vi "TraverseControl.vi"(0 "Mode":T5=enum."Read traverse position", 1 "Work in Tunnel Coordinates?":T2, 2 "Probe Support":T1=[{"Max"=15001.0, "Min"=12000.0}, {"Max"=1000.0, "Min"=-1000.0}, {"Max"=700.0, "Min"=0.0}] {"Min" format="%#.1f"; "Max" format="%#.1f"}, 3 "Model       Roll      Pitch       Yaw (deg)":dbl[](array[numeric]) format="%#.2f", 4 "Probe Volume":T1=[{"Max"=15.0, "Min"=-15.0}, {"Max"=250.0, "Min"=0.0}, {"Max"=15.0, "Min"=-15.0}] {"Min" format="%#.1f"; "Max" format="%#.1f"}, 5 "Position input XYZ":dbl[](array[numeric])=[0.0, 0.0, 0.0] format="%.2f", 6 "Route Checking?":bool, 7 "Entire Space":T1=[{"Max"=15001.0, "Min"=12000.0}, {"Max"=1000.0, "Min"=-1000.0}, {"Max"=700.0, "Min"=0.0}] {"Min" format="%#.1f"; "Max" format="%#.1f"}, 10 "Exclude Array":T3[](array[typedef]) {"Sizes"."Min" format="%#.1f"; "Sizes"."Max" format="%#.1f"}, 11 "Speed Factor":dbl=1.0 min=0.1 max=5.0 format="%.2f", 12 "Traverse Name":string, 13 "Backlash Compensation?":bool=TRUE) -> (14 "Position Output XYZ":dbl[](array[numeric]) format="%.2f", 19 "Error String":string)   [LabVIEW 2013]
uses:
  Anemometry/Anemometry Sub Vis/Gen Trav/Trav_mode.ctl
  Anemometry/Anemometry Sub Vis/Gen Trav/Route mapping/Exclude_cluster.ctl
  Anemometry/Anemometry Sub Vis/Gen Trav/Route mapping/Box_size.ctl
  Anemometry/Anemometry Sub Vis/Gen Trav/Route mapping/Exclusion_type.ctl
  Anemometry/Anemometry Sub Vis/Controls/Tunnel_Coordinates.ctl
  ~subVIs/GenericDriveCommand.ctl
  ADAM Client/Sub VIs/ADAM Controls/Update_scan_value.ctl
  Anemometry/Anemometry Sub Vis/Globals/Trav_pos_global.vi
  Anemometry/Anemometry Sub Vis/Globals/Preference_global.vi
  ~subVIs/DriveConfigGlobal.vi
panel:
  out "Server copy Location":path
  out "Position Steps":dbl[][](array[numeric]) format="%.2f"
  out "Log File":path
  out "Achieved Pos In Eng units of all channels":dbl[](array[numeric]) format="%.2f"
  out "Pulses Positon all channels":dbl[](array[numeric])
  out "Counters Reset?":bool
  # "X                Y                   Z"
  # "X                           Y                          Z"
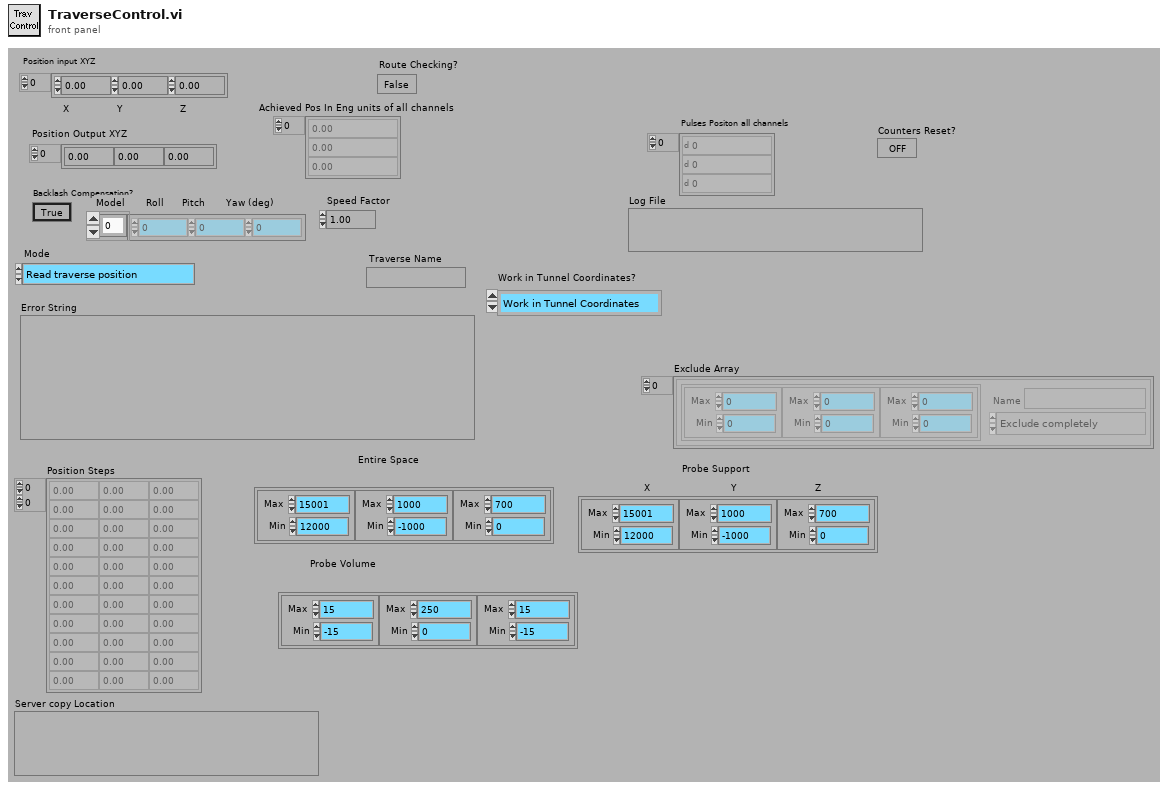
[diagram p1: front panel]
types:
  T1 = typedef "Box_size.ctl" = cluster{"Max":dbl, "Min":dbl}[]
  T2 = typedef "Tunnel_Coordinates.ctl" = enum16{"Work in Tunnel Coordinates", "Work in Model Coordinates"}
  T3 = typedef "Exclude_cluster.ctl" = cluster{"Sizes":T1, "Name":string, "Exclude Type":T4}
  T4 = typedef "Exclusion_type.ctl" = enum16{"Exclude completely", "Allow only vertical moves"}
  T5 = typedef "Trav_mode.ctl" = enum16{"Move traverse", "Read traverse position", "Teach Position"}
  T6 = typedef "GenericDriveCommand.ctl" = string
  T7 = enum16{"To Traverse Coordinates", "To User Coordinates"}
  T8 = typedef "Update_scan_value.ctl" = cluster{"Channel Name":string, "New Value":dbl}
  T9 = typedef "AxisConfigCluster.ctl" = cluster{"Channel Properties":T10, "Static Drive Configuration":T11}
  T10 = typedef "DriveProperties.ctl" = cluster{"Channel Name":string, "Vel. Default":dbl, "Acc. Default":dbl, "Vel. Max":dbl, "Vel. Min":dbl, "Acc. Max":dbl, "Acc. Min":dbl, "Pulses/unit":dbl, "Address":u8, "Pulse Offset":i32, "Pos Tolerance":dbl, "Pulses/rev":dbl, "Backlash/Eng units":dbl, "Current Pos":dbl, "Ch Status":enum16{"Active", "Offline", "Simulate"}, "Port Name":string, "Axis Transform mode":string, "Metadata Ch Name":string, "Type":string}
  T11 = typedef "DriveStaticConfig.ctl" = cluster{"Correction Gain % (CG)":u16, "Dead Band (DB)":i32, "Dead Band Window (DW)":i32, "Encoder Resolution (ER)":i32, "Step Mode  (FSB)":u16, "Position Maintenance (FSC)":u16, "Stop on Stall (FSD)":u16, "Activate OP1 on stall (FSE)":u16, "Stop on Trigger 3 (FSF)":u16, "OP2 in Deadband (FSG)":u16, "Stall Detect (FSH)":u16, "Limit Disable (LD)":u16, "Motor Resolution (MR)":enum16{"200", "400", "1000", "2000", "4000", "5000", "10000", "12800", "18000", "20000", "21600", "25000", "25400", "25600", "36000", "50000", "278528", "425984", "507904", "614400", "655360", "819200", "1024000"}, "Limit Switch Sense (OSA)":u16, "Home Position (OSB)":u16, "Home Switch Sense (OSC)":u16, "Encoder Z for Home (OSD)":u16, "Reference edge of Home (OSH)":u16, "RS232 Echo Control (SSA)":u16, "Buffer at Limit (SSG)":u16, "Buffer at Stop (SSH)":u16, "Indexer Mode  (FSA)":u16, "Type":string, "ConfigString":string, "De Power Motor":enum16{"TRUE", "FALSE"}}
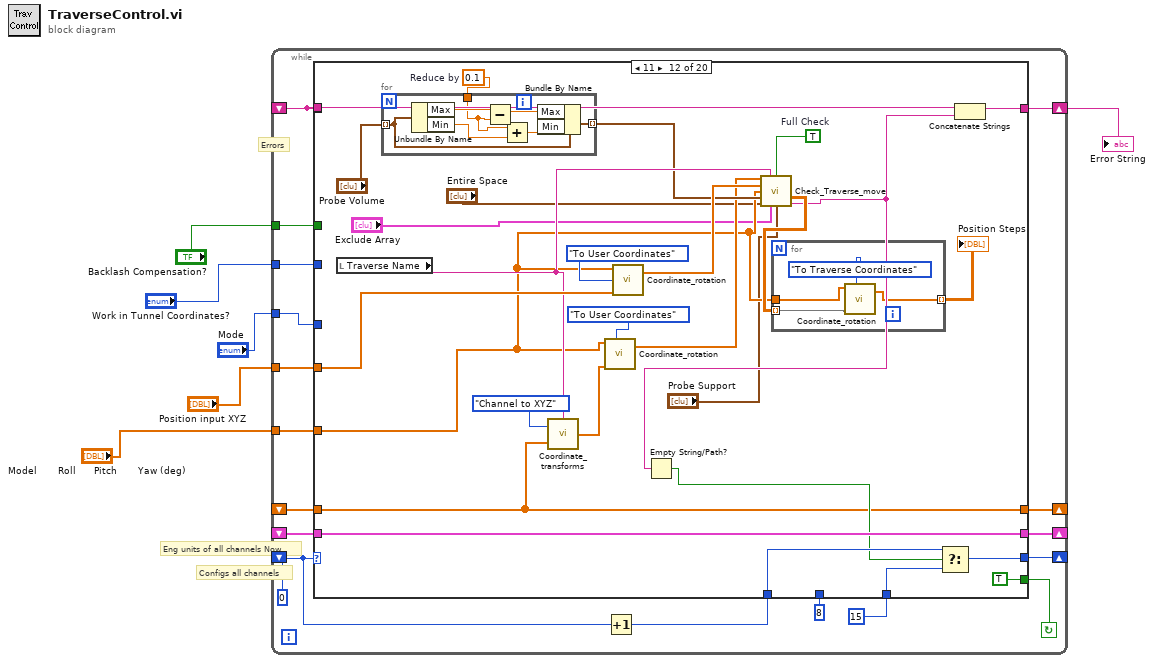
[diagram p0: block diagram]
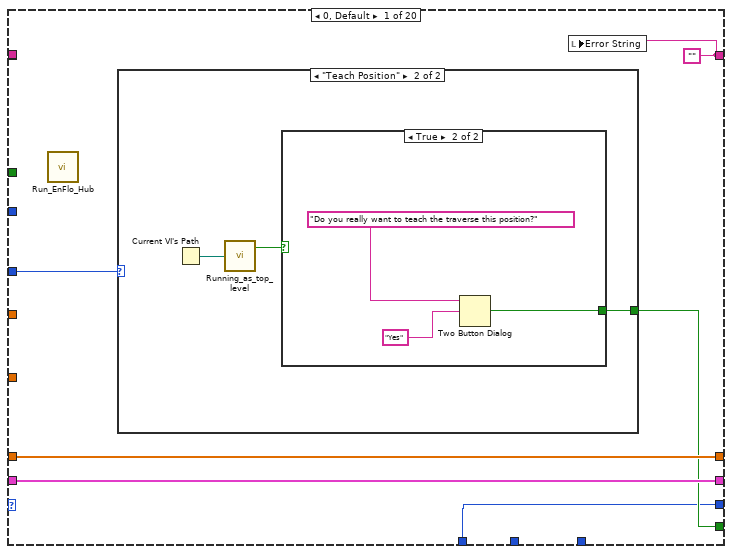
[diagram p2: hidden frame]
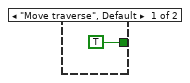
[diagram p3: hidden frame]
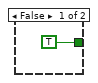
[diagram p4: hidden frame]
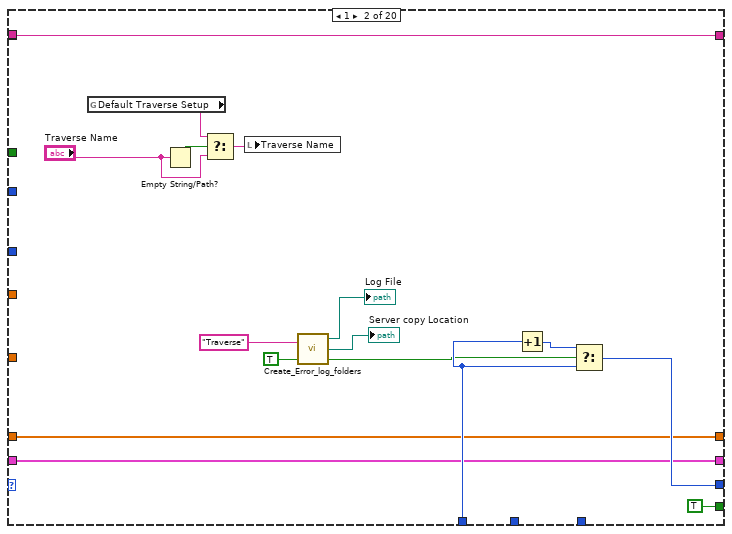
[diagram p5: hidden frame]
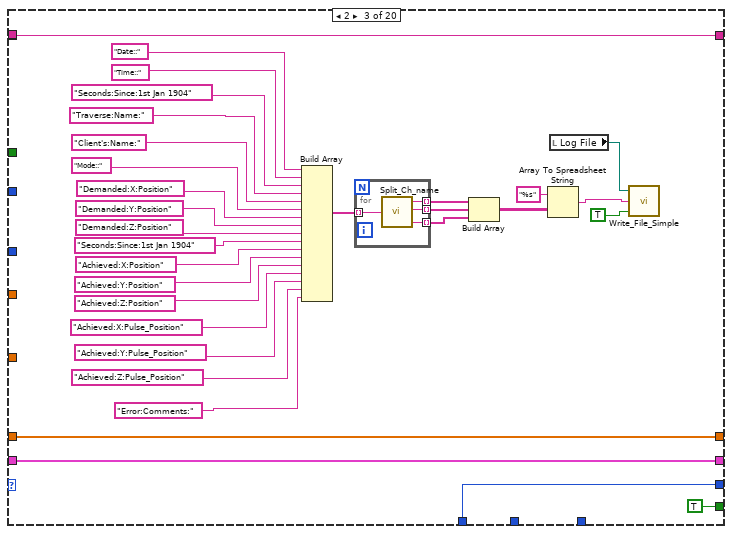
[diagram p6: hidden frame]
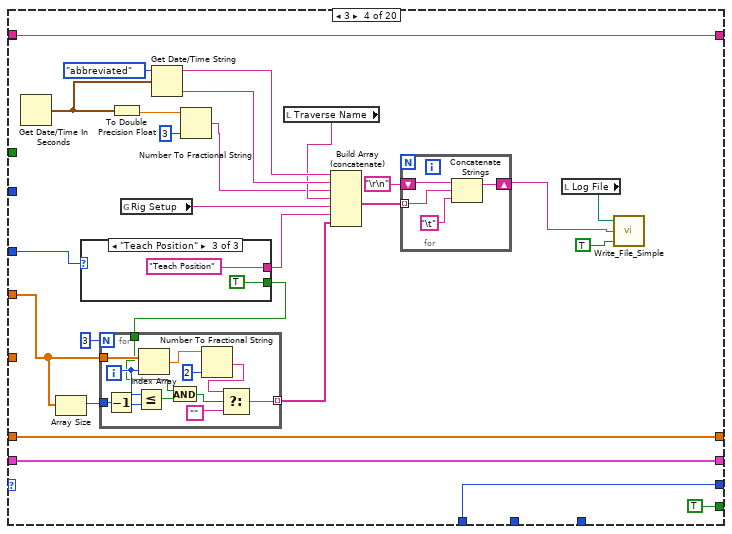
[diagram p7: hidden frame]
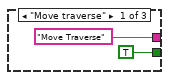
[diagram p8: hidden frame]
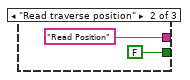
[diagram p9: hidden frame]
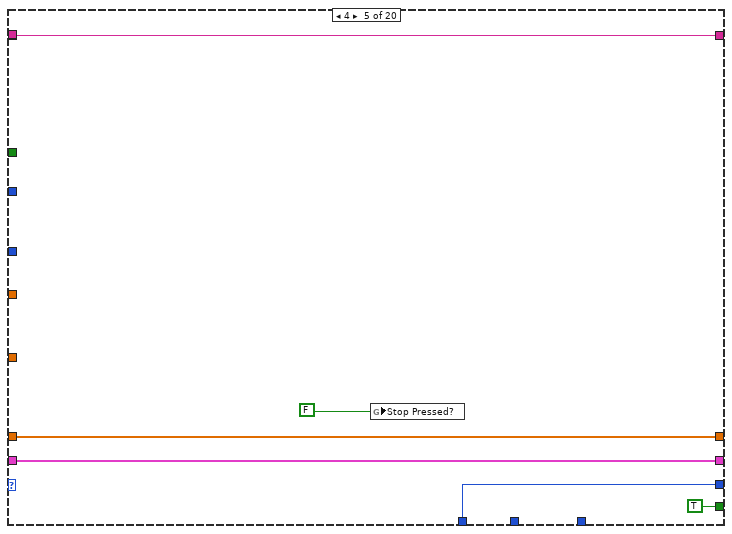
[diagram p10: hidden frame]
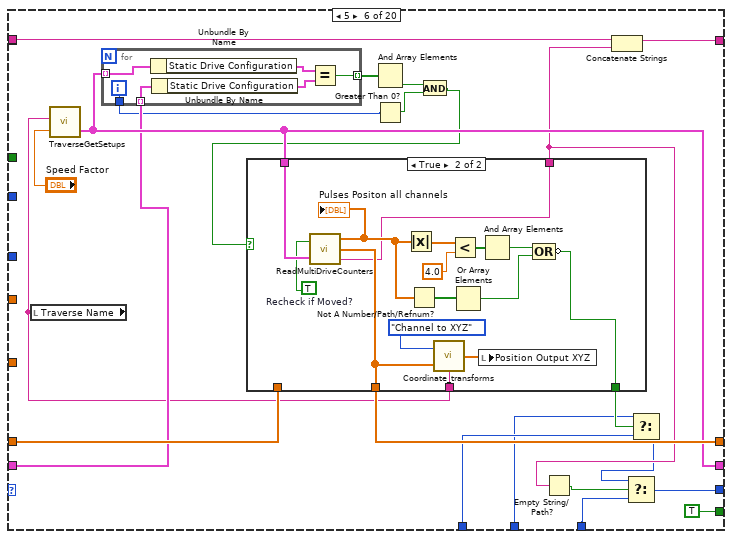
[diagram p11: hidden frame]
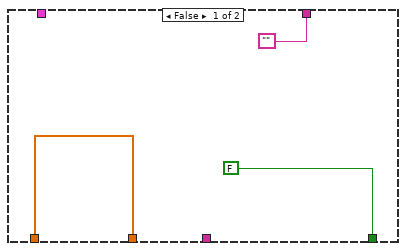
[diagram p12: hidden frame]
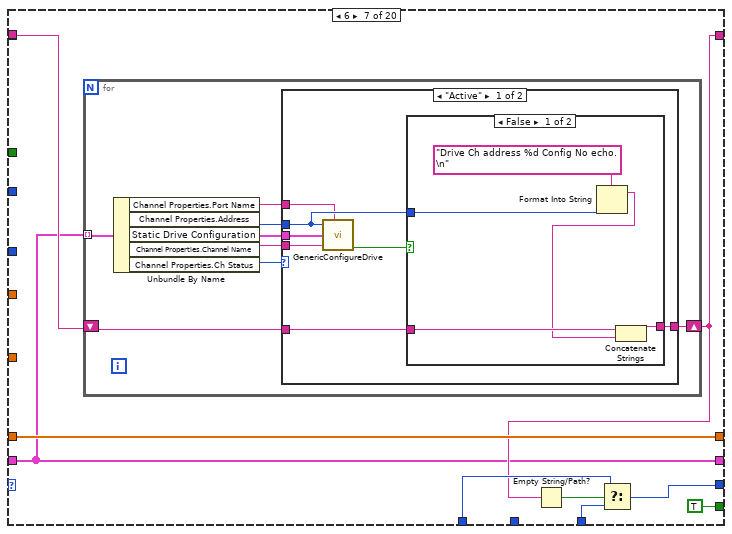
[diagram p13: hidden frame]
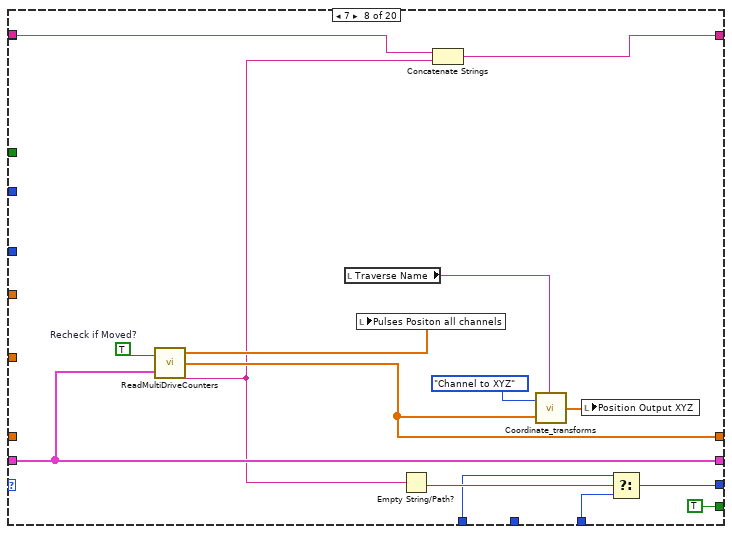
[diagram p16: hidden frame]
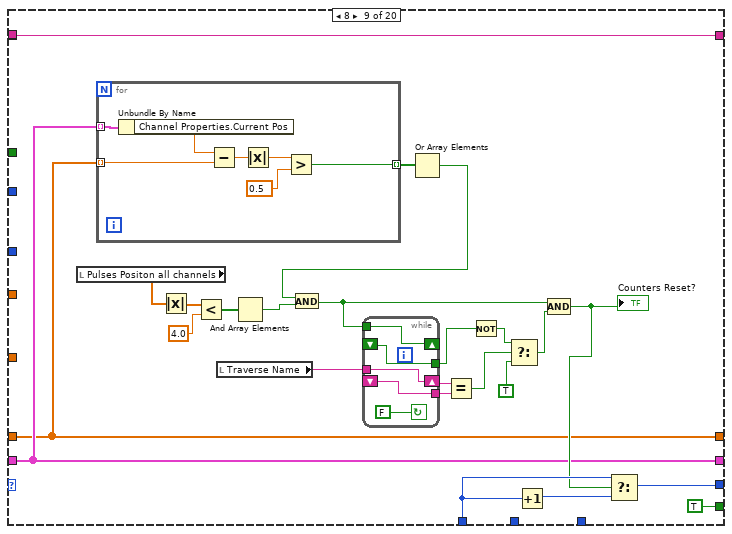
[diagram p17: hidden frame]
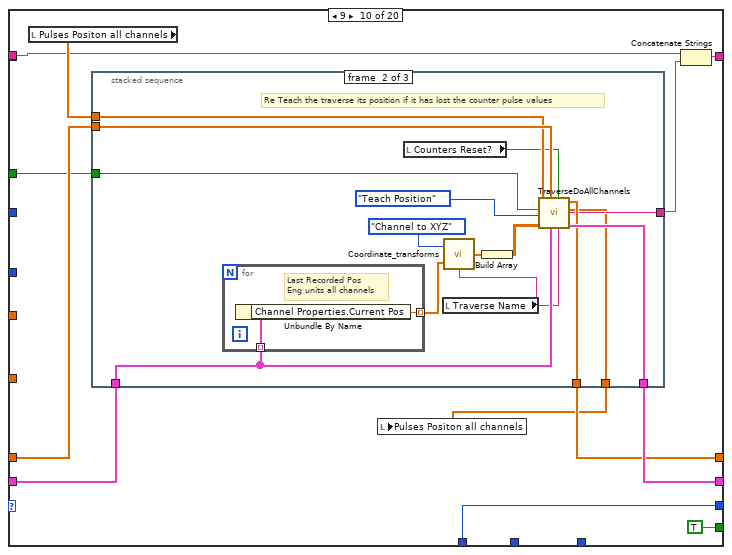
[diagram p18: hidden frame]
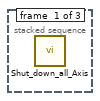
[diagram p19: hidden frame]
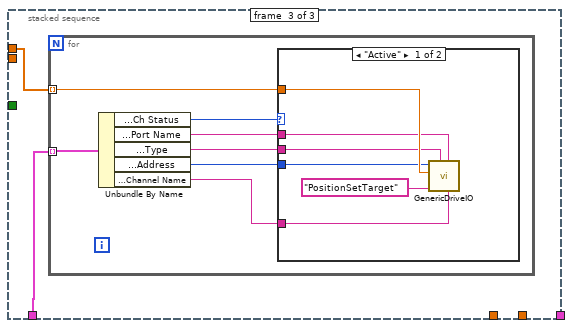
[diagram p20: hidden frame]
diagram:
  # "Errors"
  # "Eng units of all channels Now"
  # "Configs all channels"
  n1 = while {
    tunnel: "Backlash Compensation?" -> [w10]
    tunnel: "Position input XYZ" -> [w14]
    shift-left: _ -> [w11]
    shift-right: [w15] -> w5
    shift-left: _ -> [w16]
    shift-right: [w17] -> _
    shift-left: _ -> [w18]
    shift-right: [w19] -> _
    shift-left: 0 -> [w22]
    shift-right: [w20] -> _
    tunnel: "Mode" -> [w24]
    tunnel: "Model       Roll      Pitch       Yaw (deg)" -> [w9]
    tunnel: "Work in Tunnel Coordinates?" -> [w8]
    stop <- w23 continue-if-true
    n2 = Increment(x=w22) -> (x+1=w21:i32)
    n3 = case shown="11" w22 {
      tunnel: w24 -> [w30 _ _ w108 _ _ _ _ _ _ w323 _ w389 w396 _ _ _ w471 _ w527]
      tunnel: [w27 TRUE ("T button?") TRUE ("T button?") TRUE ("T button?") TRUE TRUE ("T button?") TRUE ("T button?") TRUE ("T button?") TRUE TRUE TRUE ("T button?") TRUE ("T button?") TRUE TRUE TRUE ("T button?") TRUE ("T button?") TRUE ("T button?") w473 TRUE FALSE] -> w23
      tunnel: w21 -> [w26 w53 w65 w113 w138 w162 w195 w223 w255 w274 w322 w357 w380 w398 w421 w438 w466 w470 w505 w534]
      tunnel: [w26 w51 w65 w113 w138 w145 w194 w221 w253 w274 w321 w358 w380 w397 w421 w436 w466 w469 w505 w534] -> w20
      tunnel: [w28 w48 w67 w115 w140 w160 w190 w235 w250 w283 w319 w360 w373 w395 w423 w449 w468 w476 w503 w532] -> w19
      tunnel: w18 -> [w28 w48 w67 w115 w140 w159 w190 w235 w250 w282 w319 w360 w387 w395 w423 w449 w468 w476 w503 w532]
      tunnel: [w29 w49 w66 w114 w141 w165 w198 w230 w249 w279 w318 w347 w381 w401 w422 w448 w467 w477 w506 w535] -> w17
      tunnel: w16 -> [w29 w49 w66 w114 w141 w164 w198 _ w249 w280 w318 w347 w376 w401 w422 w448 w467 w477 w506 w535]
      tunnel: [w25 w47 w63 w105 w142 w150 w191 w226 w252 w276 w324 w351 w383 w399 w419 w440 w464 w472 w499 w528] -> w15
      tunnel: w11 -> [_ w47 w63 w105 w142 w151 w192 w227 w252 w278 w324 _ w384 w399 w419 w440 w464 w475 w501 w530]
      tunnel: w14 -> [_ _ _ w102 _ _ _ _ _ _ w317 w349 _ _ _ _ _ _ w497 _]
      tunnel: 15 ("f") -> [_ _ _ _ _ w146 w193 w222 _ _ _ w353 _ _ _ _ _ _ _ _]
      tunnel: 8 ("t") -> [_ _ _ _ _ w161 _ _ _ _ _ _ _ _ _ _ _ _ _ _]
      tunnel: w11 -> [_ _ _ _ _ _ _ _ _ _ _ w354 _ _ _ _ _ _ _ _]
      tunnel: w10 -> [_ _ _ _ _ _ _ _ _ w273 _ _ w375 _ _ _ _ _ _ _]
      tunnel: w9 -> [_ _ _ _ _ _ _ _ _ _ _ w337 _ _ _ _ _ _ w498 w525]
      tunnel: w8 -> [_ _ _ _ _ _ _ _ _ _ _ _ _ _ _ _ _ _ w495 w523]
      frame 0, Default {
        w25 = ""
        n4 = call "Run_EnFlo_Hub.vi"() -> ()  [unwired: 8 out]
        n5 = case shown="\"Teach Position\"" w30 {
          tunnel: [TRUE ("T button?") w32] -> w27
          frame "Move traverse", Default {
          }
          frame "Teach Position" {
            n6 = Current VI's Path() -> (path=w34:path)
            n7 = call "Running_as_top_level.vi"("Vi path name"=w34) -> ("Top Level"=w33:bool)  [unwired: 1 out]
            n8 = case shown="True" w33 {
              tunnel: [TRUE ("T button?") w36] -> w32
              frame False {
              }
              frame True {
                n9 = Two Button Dialog(message="Do you really want to teach the traverse this position?", 2:"Yes" ("T button name (\"OK\")")) -> (T button?=w36:bool)  [unwired: 1 out]
              }
            }
          }
        }
        n10 = local write "Error String"(w25) -> ()
      }
      frame 1 {
        n11 = global read "Trav_pos_global.vi" "Default Traverse Setup"() -> (w44:string)
        n12 = Empty String/Path?(string/path="Traverse Name") -> (empty?=w42:bool)
        n13 = Select(t=w44, s=w42, f="Traverse Name") -> (s? t:f=w41:string)
        n14 = local write "Traverse Name"(w41) -> ()
        n15 = call "Create_Error_log_folders.vi"("Per Day Log File?"=TRUE, "Log Filename"="Traverse" ("Input Element")) -> ("exists?"=w45:bool, "Server copy Location"=→"Server copy Location":path, "Local Log File"=→"Log File":path)  [unwired: 1 in]
        n16 = Increment(x=w53) -> (x+1=w52:i32)
        n17 = Select(t=w52, s=w45, f=w53) -> (s? t:f=w51:i32)
      }
      frame 2 {
        n18 = Build Array("Date::", "Time::", "Seconds:Since:1st Jan 1904", "Traverse:Name:", "Client's:Name:", "Mode::", "Demanded:X:Position", "Demanded:Y:Position", "Demanded:Z:Position", "Seconds:Since:1st Jan 1904", "Achieved:X:Position", "Achieved:Y:Position", "Achieved:Z:Position", "Achieved:X:Pulse_Position", "Achieved:Y:Pulse_Position", "Achieved:Z:Pulse_Position", "Error:Comments:") -> (w70:string[])
        n19 = for {
          tunnel: w70 -> [w89] mode=indexing
          tunnel: [w88] -> w71 mode=indexing
          tunnel: [w87] -> w72 mode=indexing
          tunnel: [w86] -> w73 mode=indexing
          n20 = call "Split_Ch_name.vi"("Ch name"=w89) -> ("Top level"=w88:string, "Middle"=w87:string, "Low level"=w86:string)
        }
        n21 = Build Array(w71, w72, w73) -> (w68:string[][])
        n22 = Array To Spreadsheet String(array=w68, 3:"%s" ("format string")) -> (spreadsheet string=w61:string)  [unwired: 1 out]
        n23 = local read "Log File"() -> (w60:path)
        n24 = call "Write_File_Simple.vi"("append to file? (new file:F)"=TRUE, "character string"=w61, "file path"=w60) -> ()  [unwired: 2 out]
      }
      frame 3 {
        n25 = Get Date/Time In Seconds() -> (seconds since 1Jan1904=w94:timestamp)
        n26 = Array Size(array=w102) -> (size(s)=w103:i32)
        n27 = case shown="\"Teach Position\"" w108 {
          tunnel: ["Move Traverse" "Read Position" "Teach Position"] -> w109
          tunnel: [TRUE FALSE TRUE] -> w99
          frame "Move traverse" {
          }
          frame "Read traverse position" {
          }
          frame "Teach Position" {
          }
        }
        n28 = for {
          N: 3 -> [_]
          tunnel: w102 -> [w127]
          tunnel: w103 -> [w124]
          tunnel: [w120] -> w100 mode=indexing
          tunnel: w99 -> [w116]
          i -> [w122]
          n29 = Decrement(x=w124) -> (x-1=w123:i32)
          n30 = Less Or Equal?(x=w122, y=w123) -> (x <= y?=w118:bool)
          n31 = Index Array(array=w127, index=w122) -> (element=w126:dbl)
          n32 = And(x=w116, y=w118) -> (x .and. y?=w117:bool)
          n33 = Number To Fractional String(number=w126, precision (6)=i16 2) -> (F-format string=w121:string)  [unwired: 2 out]
          n34 = Select(t=w121, s=w117, f="") -> (s? t:f=w120:string)
        }
        n35 = To Double Precision Float(number=w94) -> (double precision float=w93:dbl)
        n36 = global read "Preference_global.vi" "Rig Setup"() -> (w90:string)
        n37 = Get Date/Time String(date format (0)=enum16{"short", "long", "abbreviated"}."abbreviated", seconds (now)=w94) -> (date string=w111:string, time string=w110:string)  [unwired: 1 out]
        n38 = Number To Fractional String(number=w93, precision (6)=i16 3) -> (F-format string=w91:string)  [unwired: 2 out]
        n39 = local read "Traverse Name"() -> (w95:string)
        n40 = Build Array (concatenate)(w111, w110, w91, w95, w90, w109, w100) -> (w106:string[])
        n41 = for {
          shift-right: [w130] -> w96
          shift-left: "\r\n" -> [w131]
          tunnel: w106 -> [w129] mode=indexing
          n42 = Concatenate Strings(w131, w129, "\t") -> (w130:string)
        }
        n43 = local read "Log File"() -> (w97:path)
        n44 = call "Write_File_Simple.vi"("append to file? (new file:F)"=TRUE, "character string"=w96, "file path"=w97) -> ()  [unwired: 2 out]
      }
      frame 4 {
        n45 = global write "DriveConfigGlobal.vi" "Stop Pressed?"(FALSE) -> ()
      }
      frame 5 {
        n46 = local read "Traverse Name"() -> (w153:string)
        n47 = call "TraverseGetSetups.vi"("Speed Factor"="Speed Factor", "Traverse Name"=w153) -> ("Matched Configurations"=w160:T9[])  [unwired: 1 out]
        n48 = for {
          tunnel: w160 -> [w171] mode=indexing
          tunnel: w159 -> [w170] mode=indexing
          tunnel: [w167] -> w158 mode=indexing
          tunnel: [w166] -> w157
          i -> [w166]
          n49 = Unbundle By Name(w171) -> ("Static Drive Configuration"=w169:T11)
          n50 = Unbundle By Name(w170) -> ("Static Drive Configuration"=w168:T11)
          n51 = Equal?(x=w169, y=w168) -> (x = y?=w167:bool)
        }
        n52 = And Array Elements(Boolean array=w158) -> (logical AND=w155:bool)
        n53 = Greater Than 0?(x=w157) -> (x > 0?=w156:bool)
        n54 = And(x=w155, y=w156) -> (x .and. y?=w154:bool)
        n55 = case shown="True" w154 {
          tunnel: w160 -> [_ w189]
          tunnel: [w174 w179] -> w165
          tunnel: w164 -> [w174 _]
          tunnel: [FALSE w181] -> w163
          tunnel: w153 -> [_ w177]
          tunnel: ["" w175] -> w149
          frame False {
          }
          frame True {
            w176 = TRUE  # Recheck if Moved?
            n56 = call "ReadMultiDriveCounters.vi"("Recheck if Moved?"=w176, "Matched Configurations"=w189) -> ("Pulses"=w184:dbl[], "Eng units"=w179:dbl[], "Error String"=w175:string)
            "Pulses Positon all channels" <- w184
            n57 = Absolute Value(x=w184) -> (abs(x)=w188:dbl[])
            n58 = Not A Number/Path/Refnum?(number/path/refnum=w184) -> (NaN/Path/Refnum?=w183:bool[])
            n59 = call "Coordinate_transforms.vi"("Traverse Name"=w177, "Input"=w179, "Mode"=enum16{"XYZ to Channel", "Channel to XYZ"}."Channel to XYZ") -> ("Output"=w178:dbl[])
            n60 = Less?(x=w188, y=4.0 ("Achieved Position")) -> (x < y?=w186:bool[])
            n61 = Or Array Elements(Boolean array=w183) -> (logical OR=w182:bool)
            n62 = local write "Position Output XYZ"(w178) -> ()
            n63 = And Array Elements(Boolean array=w186) -> (logical AND=w185:bool)
            n64 = Compound Arithmetic op=OR(w185, w182) -> (invert w181:bool)
          }
        }
        n65 = Empty String/Path?(string/path=w149) -> (empty?=w148:bool)
        n66 = Concatenate Strings(w151, w149) -> (w150:string)
        n67 = Select(t=w161, s=w163, f=w162) -> (s? t:f=w147:i32)
        n68 = Select(t=w147, s=w148, f=w146) -> (s? t:f=w145:i32)
      }
      frame 6 {
        n69 = for {
          tunnel: w190 -> [w206] mode=indexing
          shift-right: [w199] -> w191
          shift-left: w192 -> [w200]
          n70 = Unbundle By Name(w206) -> ("Channel Properties.Port Name"=w201:string, "Channel Properties.Address"=w205:u8, "Static Drive Configuration"=w204:T11, "Channel Properties.Channel Name"=w203:string, "Channel Properties.Ch Status"=w202:enum16{"Active", "Offline", "Simulate"})
          n71 = case shown="\"Active\"" w202 {
            tunnel: w205 -> [w211 _]
            tunnel: w204 -> [w213 _]
            tunnel: w203 -> [w212 _]
            tunnel: w201 -> [w210 _]
            tunnel: w200 -> [w208 w220]
            tunnel: [w207 w220] -> w199
            frame "Active" {
              n72 = call "GenericConfigureDrive.vi"("Address"=w211, "Port Name"=w210, "Static Drive Configuration"=w213, "Channel Name"=w212) -> ("Good Echo"=w209:bool)  [unwired: 4 out]
              n73 = case shown="False" w209 {
                tunnel: w211 -> [w218 _]
                tunnel: w208 -> [w216 w219]
                tunnel: [w215 w219] -> w207
                frame False {
                  n74 = Format Into String(format string="Drive Ch address %d Config No echo.\n" ("Format String"), w218) -> (resulting string=w214:string)  [unwired: 2 in, 1 out]
                  n75 = Concatenate Strings(w216, w214) -> (w215:string)
                }
                frame True {
                }
              }
            }
            frame "Offline", Default {
            }
          }
        }
        n76 = Empty String/Path?(string/path=w191) -> (empty?=w196:bool)
        n77 = Select(t=w195, s=w196, f=w193) -> (s? t:f=w194:i32)
      }
      frame 7 {
        w228 = TRUE  # Recheck if Moved?
        n78 = call "ReadMultiDriveCounters.vi"("Recheck if Moved?"=w228, "Matched Configurations"=w235) -> ("Pulses"=w233:dbl[], "Eng units"=w230:dbl[], "Error String"=w224:string)
        n79 = local read "Traverse Name"() -> (w229:string)
        n80 = local write "Pulses Positon all channels"(w233) -> ()
        n81 = Empty String/Path?(string/path=w224) -> (empty?=w225:bool)
        n82 = Concatenate Strings(w227, w224) -> (w226:string)
        n83 = call "Coordinate_transforms.vi"("Traverse Name"=w229, "Input"=w230, "Mode"=enum16{"XYZ to Channel", "Channel to XYZ"}."Channel to XYZ") -> ("Output"=w231:dbl[])
        n84 = local write "Position Output XYZ"(w231) -> ()
        n85 = Select(t=w223, s=w225, f=w222) -> (s? t:f=w221:i32)
      }
      frame 8 {
        n86 = local read "Pulses Positon all channels"() -> (w244:dbl[])
        n87 = for {
          tunnel: w250 -> [w271] mode=indexing
          tunnel: w249 -> [w269] mode=indexing
          tunnel: [w265] -> w247 mode=indexing
          n88 = Unbundle By Name(w271) -> ("Channel Properties.Current Pos"=w270:dbl)
          n89 = Subtract(x=w270, y=w269) -> (x-y=w268:dbl)
          n90 = Absolute Value(x=w268) -> (abs(x)=w267:dbl)
          n91 = Greater?(x=w267, y=0.5) -> (0:w265:bool)
        }
        n92 = Absolute Value(x=w244) -> (abs(x)=w259:dbl[])
        n93 = Less?(x=w259, y=4.0 ("Achieved Position")) -> (x < y?=w257:bool[])
        n94 = local read "Traverse Name"() -> (w243:string)
        n95 = And Array Elements(Boolean array=w257) -> (logical AND=w248:bool)
        n96 = Or Array Elements(Boolean array=w247) -> (logical OR=w246:bool)
        n97 = And(x=w246, y=w248) -> (x .and. y?=w245:bool)
        n98 = while {
          tunnel: [w263] -> w237
          tunnel: w245 -> [w264]
          shift-left: _ -> [w263]
          shift-right: [w264] -> _
          shift-right: [w261] -> w242
          shift-left: _ -> [w260]
          tunnel: w243 -> [w261]
          tunnel: [w260] -> w241
          stop <- FALSE continue-if-true
        }
        n99 = Equal?(x=w242, y=w241) -> (x = y?=w240:bool)
        n100 = Not(x=w237) -> (.not. x?=w236:bool)
        n101 = Select(t=w236, s=w240, f=TRUE) -> (s? t:f=w239:bool)
        n102 = Increment(x=w255) -> (x+1=w254:i32)
        n103 = Compound Arithmetic op=AND(w245, w239) -> (w251:bool)
        "Counters Reset?" <- w251
        n104 = Select(t=w255, s=w251, f=w254) -> (s? t:f=w253:i32)
      }
      frame 9 {
        n105 = local read "Pulses Positon all channels"() -> (w281:dbl[])
        n106 = stacked-sequence {
          tunnel: w281 -> [_ w290 w301]
          tunnel: [_ w298 _] -> w283
          tunnel: w280 -> [_ w297 _]
          tunnel: [_ w296 _] -> w279
          tunnel: w282 -> [_ w292 w302]
          tunnel: [_ w295 _] -> w277
          tunnel: w273 -> [_ w286 _]
          tunnel: [_ w284 _] -> w272
          frame #0 {
            n107 = call "Shut_down_all_Axis.vi"() -> ()  [unwired: 1 out]
          }
          frame #1 {
            # "Re Teach the traverse its position if it has lost the counter pulse values"
            n108 = for {
              tunnel: [w300] -> w291 mode=indexing
              tunnel: w292 -> [w299] mode=indexing
              # "Last Recorded Pos\nEng units all channels"
              n109 = Unbundle By Name(w299) -> ("Channel Properties.Current Pos"=w300:dbl)
            }
            n110 = local read "Counters Reset?"() -> (w288:bool)
            n111 = local read "Traverse Name"() -> (w287:string)
            n112 = call "Coordinate_transforms.vi"("Traverse Name"=w287, "Input"=w291, "Mode"=enum16{"XYZ to Channel", "Channel to XYZ"}."Channel to XYZ") -> ("Output"=w293:dbl[])
            n113 = Build Array(w293) -> (w285:dbl[][])
            n114 = call "TraverseDoAllChannels.vi"("Traverse Name"=w287, "Counters Reset?"=w288, "Matched Configurations all Channels In"=w292, "Current Pos In Eng units of all channels"=w297, "Position Steps"=w285, "Mode"=Trav_mode."Teach Position", "Backlash Compensation?"=w286, "Current Pulses positions for all channels"=w290) -> ("Matched Configurations Out"=w298:T9[], "Error String"=w295:string, "Current Pulses positions for all channels Out"=w284:dbl[], "Achieved Pos In Eng units of all channels"=w296:dbl[])
          }
          frame #2 {
            n115 = for {
              tunnel: w302 -> [w309] mode=indexing
              tunnel: w301 -> [w308] mode=indexing
              n116 = Unbundle By Name(w309) -> ("Channel Properties.Ch Status"=w307:enum16{"Active", "Offline", "Simulate"}, "Channel Properties.Port Name"=w306:string, "Channel Properties.Type"=w305:string, "Channel Properties.Address"=w304:u8, "Channel Properties.Channel Name"=w303:string)
              n117 = case shown="\"Active\"" w307 {
                tunnel: w308 -> [w315 _]
                tunnel: w306 -> [w314 _]
                tunnel: w305 -> [w313 _]
                tunnel: w304 -> [w312 _]
                tunnel: w303 -> [w311 _]
                frame "Active" {
                  n118 = call "GenericDriveIO.vi"("GenericDriveCommand"=T6 "PositionSetTarget", "Channel Name"=w311, "Numeric Value"=w315, "Address"=w312, "Type"=w313, "Port Name"=w314) -> ()  [unwired: 1 in, 5 out]
                }
                frame "Offline", Default {
                }
              }
            }
          }
        }
        n119 = local write "Pulses Positon all channels"(w272) -> ()
        n120 = Concatenate Strings(w278, w277) -> (w276:string)
      }
      frame 10 {
        n121 = Build Array(w317) -> (w316:dbl[][])
        n122 = local write "Position Steps"(w316) -> ()
        n123 = case shown="\"Read traverse position\", Default" w323 {
          tunnel: w322 -> [w325 w332]
          tunnel: [w327 w331] -> w321
          frame "Move traverse" {
            n124 = Increment(x=w325) -> (x+1=w326:i32)
            n125 = case shown="True" "Route Checking?" {
              tunnel: [w329 w330] -> w327
              tunnel: w326 -> [w329 _]
              tunnel: w325 -> [_ w330]
              frame False {
              }
              frame True {
              }
            }
          }
          frame "Read traverse position", Default {
            n126 = Increment(x=w332) -> (x+1=w331:i32)
          }
        }
      }
      frame 11 {
        w342 = 0.1  # Reduce by
        w346 = TRUE  # Full Check
        n127 = local read "Traverse Name"() -> (w348:string)
        n128 = for {
          tunnel: "Probe Volume" -> [w367] mode=indexing
          tunnel: [w366] -> w341 mode=indexing
          tunnel: w342 -> [w361]
          n129 = Unbundle By Name(w367) -> ("Max"=w365:dbl, "Min"=w363:dbl)
          n130 = Subtract(x=w365, y=w361) -> (x-y=w364:dbl)
          n131 = Add(x=w361, y=w363) -> (x+y=w362:dbl)
          n132 = Bundle By Name(cluster=w367, "Max"=w364, "Min"=w362) -> (w366:cluster{"Max":dbl, "Min":dbl})
        }
        n133 = call "Coordinate_transforms.vi"("Traverse Name"=w348, "Input"=w347, "Mode"=enum16{"XYZ to Channel", "Channel to XYZ"}."Channel to XYZ") -> ("Output"=w339:dbl[])
        n134 = call "Coordinate_rotation.vi"("Model       Roll      Pitch       Yaw (deg)"=w337, "Input Position"=w339, "Mode"=T7."To User Coordinates") -> ("Output Position"=w338:dbl[])  [unwired: 2 in, 1 out]
        n135 = call "Coordinate_rotation.vi"("Model       Roll      Pitch       Yaw (deg)"=w337, "Input Position"=w349, "Mode"=T7."To User Coordinates") -> ("Output Position"=w355:dbl[])  [unwired: 2 in, 1 out]
        n136 = call "Check_Traverse_move.vi"("Current position"=w338, "Traverse Name"=w348, "Full Check"=w346, "New Position"=w355, "Model       Roll      Pitch       Yaw (deg)"=w337, "Probe Volume"=w341, "Entire Space"="Entire Space", "Exclude Array"="Exclude Array", "Probe Support"="Probe Support") -> ("Steps"=w345:dbl[][], "Error Comments"=w343:string)  [unwired: 5 out]
        n137 = Empty String/Path?(string/path=w343) -> (empty?=w352:bool)
        n138 = for {
          tunnel: w345 -> [w370] mode=indexing
          tunnel: [w369] -> w344 mode=indexing
          tunnel: w337 -> [w368]
          n139 = call "Coordinate_rotation.vi"("Model       Roll      Pitch       Yaw (deg)"=w368, "Input Position"=w370, "Mode"=T7."To Traverse Coordinates") -> ("Output Position"=w369:dbl[])  [unwired: 2 in, 1 out]
        }
        "Position Steps" <- w344
        n140 = Select(t=w357, s=w352, f=w353) -> (s? t:f=w358:i32)
        n141 = Concatenate Strings(w354, w343) -> (w351:string)
      }
      frame 12 {
        w378 = FALSE  # Counters Reset?
        n142 = local read "Pulses Positon all channels"() -> (w388:dbl[])
        n143 = local read "Traverse Name"() -> (w377:string)
        n144 = local read "Position Steps"() -> (w374:dbl[][])
        n145 = call "TraverseDoAllChannels.vi"("Traverse Name"=w377, "Counters Reset?"=w378, "Matched Configurations all Channels In"=w387, "Current Pos In Eng units of all channels"=w376, "Position Steps"=w374, "Mode"=w389, "Backlash Compensation?"=w375, "Current Pulses positions for all channels"=w388) -> ("Matched Configurations Out"=w373:T9[], "Error String"=w382:string, "Current Pulses positions for all channels Out"=w372:dbl[], "Achieved Pos In Eng units of all channels"=w381:dbl[])
        "Achieved Pos In Eng units of all channels" <- w381
        n146 = call "Coordinate_transforms.vi"("Traverse Name"=w377, "Input"=w381, "Mode"=enum16{"XYZ to Channel", "Channel to XYZ"}."Channel to XYZ") -> ("Output"=→"Position Output XYZ":dbl[])
        n147 = local write "Pulses Positon all channels"(w372) -> ()
        n148 = Concatenate Strings(w384, w382) -> (w383:string)
      }
      frame 13 {
        n149 = local read "Position Output XYZ"() -> (w393:dbl[])
        n150 = case shown="\"Teach Position\"" w396 {
          tunnel: w393 -> [_ w417 _]
          frame "Move traverse" {
          }
          frame "Read traverse position" {
            n151 = local write "Position input XYZ"(w417) -> ()
          }
          frame "Teach Position" {
            n152 = local write "Mode"(Trav_mode."Teach Position" ("Mode")) -> ()
          }
        }
        n153 = for {
          tunnel: w395 -> [w409] mode=indexing
          tunnel: T8 {"Channel Name"="", "New Value"=0.0} ("Update Scan Value Cluster") -> [w408]
          tunnel: w393 -> [w406] mode=indexing
          shift-right: [w404] -> w391
          shift-left: T8[] [] -> [w405]
          n154 = Unbundle By Name(w409) -> ("Channel Properties.Metadata Ch Name"=w407:string)
          n155 = Empty String/Path?(string/path=w407) -> (empty?=w403:bool)
          n156 = case shown="False" w403 {
            tunnel: w408 -> [w415 _]
            tunnel: w407 -> [w414 _]
            tunnel: w406 -> [w413 _]
            tunnel: w405 -> [w411 w416]
            tunnel: [w410 w416] -> w404
            frame False {
              n157 = Bundle By Name(cluster=w415, "Channel Name"=w414, "New Value"=w413) -> (w412:T8)
              n158 = Build Array (concatenate)(w411, w412) -> (w410:T8[])
            }
            frame True {
            }
          }
        }
        n159 = global write "DriveConfigGlobal.vi" "Run Emergency stop loop"(FALSE ("Run Emergency stop loop")) -> ()
        n160 = Increment(x=w398) -> (x+1=w397:i32)
        n161 = call "Update_Current_Value_client.vi"("Don't Bother with check?"=FALSE, "Update array in"=w391) -> ()
      }
      frame 14 {
      }
      frame 15 {
        n162 = local read "Pulses Positon all channels"() -> (w426:dbl[])
        n163 = local read "Position Output XYZ"() -> (w425:dbl[])
        n164 = Get Date/Time In Seconds() -> (seconds since 1Jan1904=w435:timestamp)
        n165 = To Double Precision Float(number=w435) -> (double precision float=w428:dbl)
        n166 = Number To Fractional String(number=w428, precision (6)=i16 3) -> (F-format string=w427:string)  [unwired: 2 out]
        n167 = call "Remove_unprintable_Char.vi"("Input String"=w440) -> ("Output String"=w441:string)
        n168 = Build Array (concatenate)(w425, w426) -> (w424:dbl[])
        n169 = Array Size(array=w424) -> (size(s)=w443:i32)
        n170 = for {
          N: 6 -> [_]
          tunnel: w424 -> [w463]
          tunnel: w443 -> [w460]
          tunnel: [w455] -> w442 mode=indexing
          i -> [w458]
          n171 = Decrement(x=w460) -> (x-1=w459:i32)
          n172 = Less Or Equal?(x=w458, y=w459) -> (x <= y?=w457:bool)
          n173 = Index Array(array=w463, index=w458) -> (element=w462:dbl)
          n174 = Number To Fractional String(number=w462, precision (6)=i16 2) -> (F-format string=w456:string)  [unwired: 2 out]
          n175 = Select(t=w456, s=w457, f="") -> (s? t:f=w455:string)
        }
        n176 = Build Array (concatenate)(w427, w442, w441) -> (w445:string[])
        n177 = local read "Route Checking?"() -> (w439:bool)
        n178 = for {
          shift-right: [w452] -> w432
          shift-left: "" -> [w453]
          tunnel: w445 -> [w451] mode=indexing
          n179 = Concatenate Strings(w453, w451, "\t") -> (w452:string)
        }
        n180 = Increment(x=w438) -> (x+1=w437:i32)
        n181 = local read "Log File"() -> (w433:path)
        n182 = local read "Server copy Location"() -> (w430:path)
        n183 = Select(t=w437, s=w439, f=w438) -> (s? t:f=w436:i32)
        n184 = call "Write_File_Simple.vi"("append to file? (new file:F)"=TRUE, "character string"=w432, "file path"=w433) -> ("file path Out"=w431:path)  [unwired: 1 out]
        n185 = call "Updated_File_Copy.vi"("Target Path"=w430, "Source Path"=w431) -> ()  [unwired: 2 out]
      }
      frame 16 {
      }
      frame 17 {
        n186 = local read "Position Output XYZ"() -> (w478:dbl[])
        n187 = local read "Counters Reset?"() -> (w479:bool)
        n188 = Index Array(array=w478, index=2) -> (element=w484:dbl)
        n189 = Index Array(array=w478, index=0) -> (element=w486:dbl)
        n190 = Index Array(array=w478, index=1) -> (element=w485:dbl)
        n191 = Format Into String(format string="X= %.2f\tY= %.2f\tZ= %.2f" ("Format String"), w486, w485, w484) -> (resulting string=w487:string)  [unwired: 2 in, 1 out]
        n192 = case shown="\"Read traverse position\"" w471 {
          tunnel: w470 -> [w491 w493]
          tunnel: [w491 w492] -> w469
          frame "Move traverse", Default {
          }
          frame "Read traverse position" {
            n193 = Increment(x=w493) -> (x+1=w492:i32)
          }
        }
        n194 = Select(t="\nThe traverse was probably powered down since the last move. Its position has now been retaught and now all should be well.", s=w479, f="") -> (s? t:f=w480:string)
        n195 = call "Write_out_serial_log.vi"("Header message"=w487) -> ()
        n196 = Concatenate Strings(w475, w480) -> (w472:string)
        n197 = Empty String/Path?(string/path=w472) -> (empty?=w474:bool)
        n198 = Not(x=w474) -> (.not. x?=w473:bool)
      }
      frame 18 {
        # "Add demanded position"
        n199 = case shown="\"Work in Model Coordinates\"" w495 {
          tunnel: w498 -> [_ w513]
          tunnel: w497 -> [w508 w512]
          tunnel: [w508 w510] -> w496
          tunnel: [" (Tunnel Coordinates)" " (Model Coordinates)"] -> w494
          frame "Work in Tunnel Coordinates" {
          }
          frame "Work in Model Coordinates" {
            n200 = call "Coordinate_rotation.vi"("Model       Roll      Pitch       Yaw (deg)"=w513, "Input Position"=w512, "Mode"=T7."To User Coordinates") -> ("Output Position"=w510:dbl[])  [unwired: 2 in, 1 out]
          }
        }
        n201 = for {
          tunnel: w503 -> [w521] mode=indexing
          shift-right: [w516] -> w500
          shift-left: "\nDem Pos " -> [w519]
          tunnel: w496 -> [w514] mode=indexing
          n202 = Unbundle By Name(w521) -> ("Channel Properties.Channel Name"=w520:string)
          n203 = call "Split_Ch_name.vi"("Ch name"=w520) -> ("Low level"=w518:string)  [unwired: 2 out]
          n204 = Format Into String(format string="%s=%.1f, " ("Format String"), w518, w514) -> (resulting string=w515:string)  [unwired: 2 in, 1 out]
          n205 = Concatenate Strings(w519, w515) -> (w516:string)
        }
        n206 = Concatenate Strings(w501, w500, w494) -> (w499:string)
      }
      frame 19 {
        # "Add Achieved Position"
        n207 = local read "Position Output XYZ"() -> (w522:dbl[])
        n208 = case shown="\"Work in Model Coordinates\"" w523 {
          tunnel: w525 -> [_ w539]
          tunnel: [w536 w538] -> w524
          tunnel: w522 -> [w536 w537]
          frame "Work in Tunnel Coordinates" {
          }
          frame "Work in Model Coordinates" {
            n209 = call "Coordinate_rotation.vi"("Model       Roll      Pitch       Yaw (deg)"=w539, "Input Position"=w537, "Mode"=T7."To User Coordinates") -> ("Output Position"=w538:dbl[])  [unwired: 2 in, 1 out]
          }
        }
        n210 = for {
          tunnel: w532 -> [w551] mode=indexing
          shift-right: [w546] -> w529
          shift-left: "\nAchieved Pos " -> [w549]
          tunnel: w524 -> [w544] mode=indexing
          n211 = Unbundle By Name(w551) -> ("Channel Properties.Channel Name"=w550:string)
          n212 = call "Split_Ch_name.vi"("Ch name"=w550) -> ("Low level"=w548:string)  [unwired: 2 out]
          n213 = Format Into String(format string="%s=%.1f, " ("Format String"), w548, w544) -> (resulting string=w545:string)  [unwired: 2 in, 1 out]
          n214 = Concatenate Strings(w549, w545) -> (w546:string)
        }
        n215 = case shown="\"Move traverse\"" w527 {
          tunnel: ["When requesting a move." "When reading position." "When teaching position."] -> w526
          frame "Move traverse" {
          }
          frame "Read traverse position" {
          }
          frame "Teach Position" {
          }
        }
        n216 = Concatenate Strings(w530, w529, w526) -> (w528:string)
      }
    }
  }
  "Error String" <- w5
